vi "_Raise Client Certificate Requested.vi"(4 "WebView2.lvlib:WebView2 Control.lvclass":refnum<class "WebView2 Control.lvclass">, 5 "Event Data":cluster{"sender":refnum<k24>, "e":refnum<k24>}, 6 "Control Ref":refnum<k24>, 7 "Event Common Data":T1) -> ()   [LabVIEW 2025, in "WebView2.lvlib" / "WebView2 Control.lvclass"]
uses:
  WebView2 Control.lvclass
  WebView2 Control.lvclass/WebView2 Control.ctl
  Client Certificate Requested Event Data.ctl
  E:/Labview/LV 2023/PPL/PPL Builder/Libs/LV-WebView2/Source/Libs/Microsoft.Web.WebView2.Core.dll
  Libs/Microsoft.Web.WebView2.Core.dll
  WebView2 Event Filter Interface/WebView2 Event Filter Interface.lvclass
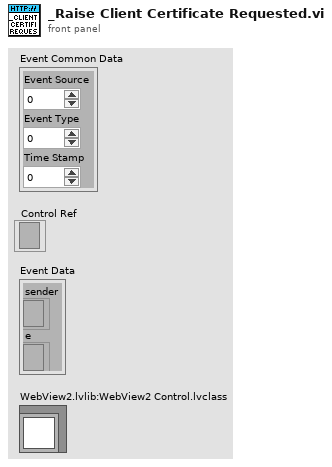
[diagram p1: front panel]
types:
  T1 = cluster{"Event Source":i32, "Event Type":u32, "Time Stamp":u32}
  T2 = typedef "WebView2.lvlib/WebView2 Control.lvclass/Client Certificate Requested Event Data.ctl" = cluster{"Host":string, "Port":i32, "IsProxy":bool, "AllowedCertificateAuthorities":refnum<k24>, "MutuallyTrustedCertificates":refnum<k24>}
  T3 = cluster{"Cancel":bool, "Handled":bool, "SelectedCertificate":refnum<k24>}
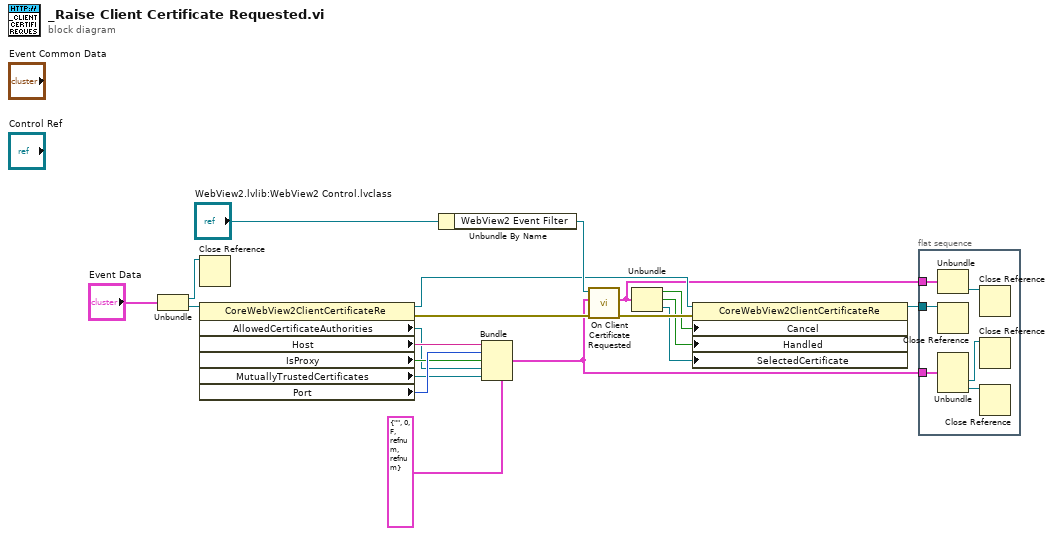
[diagram p0: block diagram]
diagram:
  n1 = Unbundle("Event Data") -> ("sender"=w19:refnum<k24>, "e"=w18:refnum<k24>)
  n2 = Close Reference(reference=w19) -> ()  [unwired: 1 in, 1 out]
  n3 = property class="CoreWebView2ClientCertificateRe"(reference=w18) -> (reference out=w10:refnum<k24>, error out=w13:errorcluster, "AllowedCertificateAuthorities"=w4:refnum<k24>, "Host"=w17:string, "IsProxy"=w15:bool, "MutuallyTrustedCertificates"=w3:refnum<k24>, "Port"=w16:i32)  [unwired: 1 in]
  n4 = Unbundle By Name("WebView2.lvlib:WebView2 Control.lvclass") -> ("WebView2 Event Filter"=w11:refnum<class "WebView2 Event Filter Interface.lvclass">)
  n5 = Bundle(cluster=T2 {"Host"="", "Port"=0, "IsProxy"=FALSE, "AllowedCertificateAuthorities"=refnum, "MutuallyTrustedCertificates"=refnum}, "Host"=w17, "Port"=w16, "IsProxy"=w15, "AllowedCertificateAuthorities"=w4, "MutuallyTrustedCertificates"=w3) -> (w2:T2)
  n6 = call-dynamic "On Client Certificate Requested.vi"("error in (no error)"=w13, "cluster"=w2, "WebView2 Event Filter Interface in"=w11) -> ("error out"=w9:errorcluster, "Response"=w1:T3)  [unwired: 7 in]
  n7 = Unbundle(w1) -> ("Cancel"=w8:bool, "Handled"=w7:bool, "SelectedCertificate"=w5:refnum<k24>)
  n8 = property class="CoreWebView2ClientCertificateRe"(reference=w10, error in=w9, "Cancel"=w8, "Handled"=w7, "SelectedCertificate"=w5) -> (reference out=w6:refnum<k24>)  [unwired: 1 out]
  n9 = flat-sequence {
    tunnel: w6 -> [w26]
    tunnel: w2 -> [w25]
    tunnel: w1 -> [w22]
    frame #0 {
      n10 = Unbundle(w22) -> ("SelectedCertificate"=w21:refnum<k24>)  [unwired: 2 out]
      n11 = Close Reference(reference=w26) -> ()  [unwired: 1 in, 1 out]
      n12 = Unbundle(w25) -> ("AllowedCertificateAuthorities"=w24:refnum<k24>, "MutuallyTrustedCertificates"=w23:refnum<k24>)  [unwired: 3 out]
      n13 = Close Reference(reference=w21) -> ()  [unwired: 1 in, 1 out]
      n14 = Close Reference(reference=w24) -> ()  [unwired: 1 in, 1 out]
      n15 = Close Reference(reference=w23) -> ()  [unwired: 1 in, 1 out]
    }
  }
